vi "PicohrdlGetSingleValue.vi"(6 "Single Ended":i16 min=0 max=1 step=1, 7 "Channel in":i16=1 min=1 max=16 step=1, 8 "error in (no error)":errorcluster, 9 "Conversion":i16 min=0 max=5 step=1, 10 "Voltage Range in":i16 min=0 max=6 step=1, 11 "handle in":i16) -> (0 "error out":errorcluster, 2 "value":i16, 3 "Handle out":i16, 4 "Over Voltage":i16)   [LabVIEW 2010]
doc: "Calls HRDLGetSingleValue()"
uses:
  PicoHRDL.dll
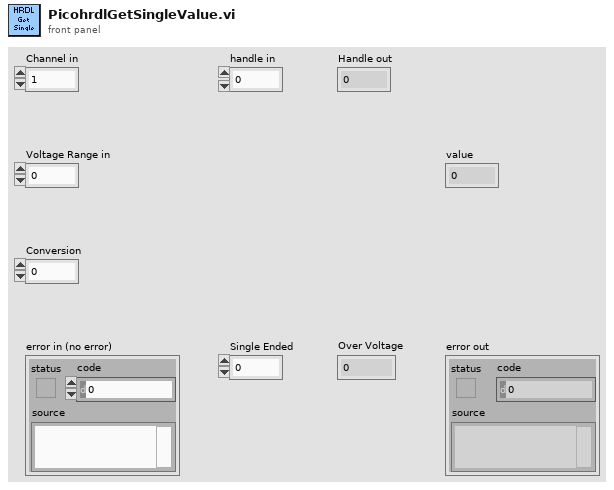
[diagram p1: front panel]
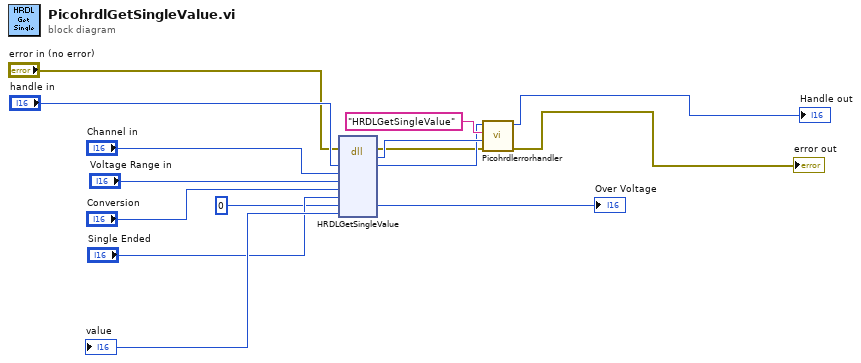
[diagram p0: block diagram]
diagram:
  n1 = dll-call lib="PicoHRDL.dll" fn="HRDLGetSingleValue"(error in="error in (no error)", "handle"="handle in", "channel"="Channel in", "range"="Voltage Range in", "conversionTime"="Conversion", "singleEnded"="Single Ended", "overflow"=i16 0) -> (error out=w10:errorcluster, "return type"=w12:i16, "handle"=w11:i16, "overflow"=→"Over Voltage":i16, "value"=→"value":i32)  [unwired: 7 in, 1 out]
  n2 = call "Picohrdlerrorhandler.vi"("Handle in"=w11, "API function"="HRDLGetSingleValue", "Return"=w12, "error in (no error)"=w10) -> ("Handle out"=→"Handle out":i16, "error out"=→"error out":errorcluster)  [unwired: 5 in]
